vi "Camera.vi"(11 "error in (no error)":errorcluster) -> (0 "Time Out (ms) 2":u8, 1 "Camera 2":bool, 2 "Feature name":string, 3 "Out":bool)   [LabVIEW 2015]
uses:
  Control Button/Exit.ctl
  Control PB/Next_.ctl
panel:
  in  "Camera":bool
  in  "Time Out (ms)":u8
  in  "Feature list":string(combo)="CAM1"
  in  "Next":T1
  in  "Exit":T2
  # "Add Feature List"
  # "CAM1"
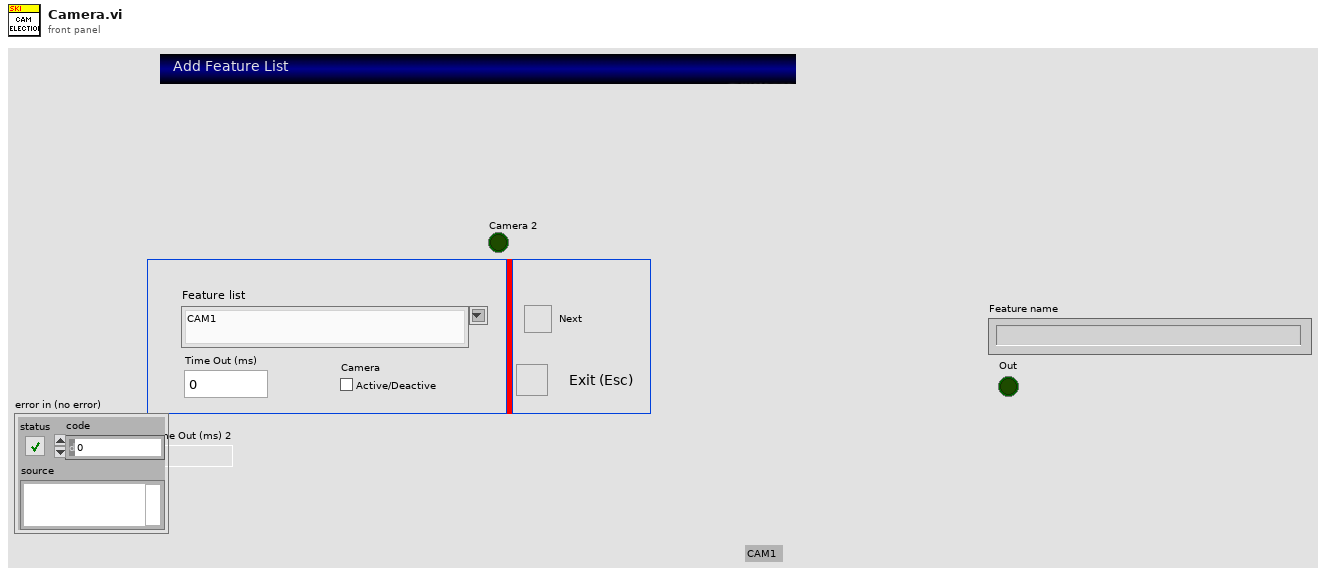
[diagram p1: front panel]
types:
  T1 = typedef "Next_.ctl" = bool
  T2 = typedef "Exit.ctl" = bool
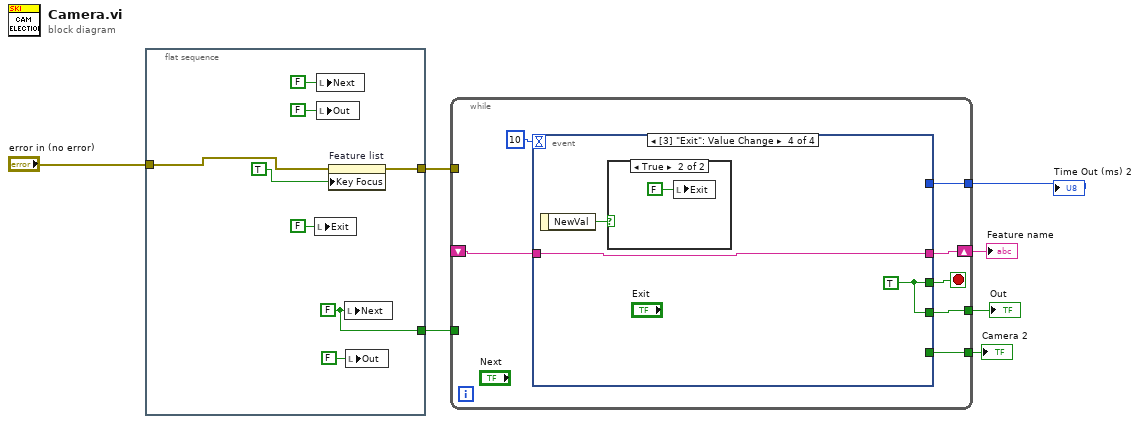
[diagram p0: block diagram]
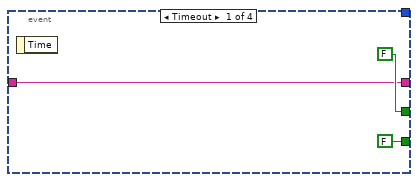
[diagram p2: hidden frame]
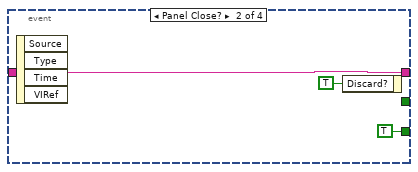
[diagram p3: hidden frame]
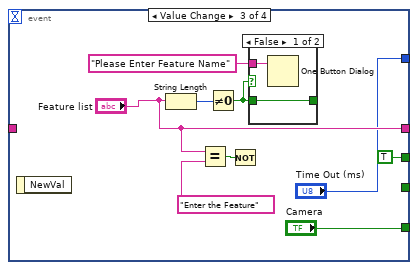
[diagram p4: hidden frame]
diagram:
  n1 = flat-sequence {
    tunnel: [w12] -> w5
    tunnel: [w9] -> w4
    tunnel: "error in (no error)" -> [w8]
    frame #0 {
      w12 = T1 FALSE ("Next")
      n2 = local write "Exit"(FALSE ("Exit")) -> ()
      n3 = local write "Next"(T1 FALSE ("Next")) -> ()
      n4 = local write "Out"(FALSE ("Out")) -> ()
      n5 = property on="Feature list" class="CmbBox"(error in=w8, "Key Focus"=TRUE) -> (error out=w9:errorcluster)  [unwired: 1 in, 1 out]
      n6 = local write "Next"(w12) -> ()
      n7 = local write "Out"(FALSE ("Out")) -> ()
    }
  }
  n8 = while {
    tunnel: [w20] -> w6
    tunnel: w5 -> [_]
    shift-right: [w21] -> w7
    shift-left: _ -> [w18]
    tunnel: w4 -> [_]
    tunnel: [w17] -> w3
    tunnel: [w16] -> w2
    stop <- w22 stop-if-true
    n9 = event shown="[3] \"Exit\": Value Change" {
      selector: _ -> [_ _ _ _]
      dyn-events: _ -> [_ _ _ _]
      timeout: 10 -> [_ _ _ _]
      tunnel: [FALSE _ TRUE w41] -> w22
      tunnel: [w23 w26 "Feature list" w42] -> w21
      tunnel: [T1 FALSE ("NewVal") T1 TRUE ("NewVal") _ w41] -> w20
      tunnel: w18 -> [w23 w26 _ w42]
      tunnel: [_ _ "Time Out (ms)" _] -> w17
      tunnel: [_ _ "Camera" _] -> w16
      event Timeout {
        n10 = event-data() -> ()  [unwired: 1 in, 1 out]
      }
      event Panel Close? {
        n11 = event-data() -> ()  [unwired: 1 in, 4 out]
        n12 = event-data("Discard?"=TRUE) -> ()  [unwired: 1 in, 1 out]
      }
      event Value Change {
        n13 = event-data() -> ()  [unwired: 1 in, 1 out]
        n14 = String Length(string="Feature list") -> (length=w37:i32)
        n15 = Equal?(x="Feature list", y="Enter the Feature") -> (x = y?=w33:bool)
        n16 = Not Equal To 0?(x=w37) -> (x != 0?=w35:bool)
        n17 = Not(x=w33) -> ()  [unwired: 1 out]
        n18 = case shown="False" w35 {
          tunnel: "Please Enter Feature Name" ("message") -> [w39 _]
          tunnel: [w38 w40] -> _
          tunnel: w35 -> [w38 w40]
          frame False {
            n19 = One Button Dialog(message=w39) -> ()  [unwired: 1 in, 1 out]
          }
          frame True {
          }
        }
      }
      event Value Change {
        w41 = TRUE
        n20 = event-data() -> ("NewVal"=w43:T2)  [unwired: 1 in]
        n21 = case shown="True" w43 {
          frame False {
          }
          frame True {
            n22 = local write "Exit"(T1 FALSE ("Next")) -> ()
          }
        }
      }
    }
  }
  "Feature name" <- w7
  "Out" <- w6
  "Time Out (ms) 2" <- w3
  "Camera 2" <- w2
